vi "Antenna_in.vi"(6 "Store":T1=enum."in_up", 8 "error in (no error)":errorcluster, 10 "Waveform in":waveform(dbl), 11 "RFID system in":refnum<class "RFID system.lvclass">) -> (0 "error out":errorcluster, 2 "Waveform out":waveform(dbl), 3 "RFID system out":refnum<class "RFID system.lvclass">)   [LabVIEW 2019, in "RFID system.lvclass"]
uses:
  RFID system.lvclass
  TypeDef/Store.ctl
  <vilib>/measure/macond.llb/IIR Filter for 1 Chan.vi
  <vilib>/measure/NI_MAPro.lvlib
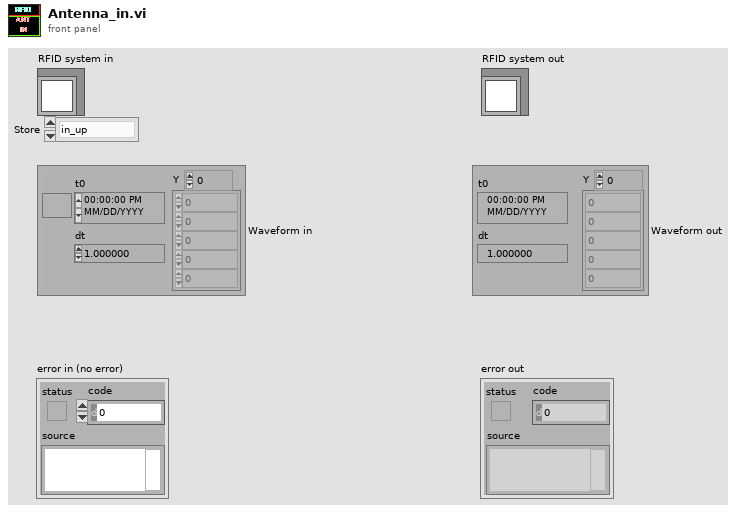
[diagram p1: front panel]
types:
  T1 = typedef "Store.ctl" = enum16{"envelope", "noise", "demSubCar", "CH_frame", "Decode", "demodulate", "in", "out", "sum", "subCarrier", "frame", "command", "encode", "modulate", "encode_UP", "modulate_up", "demod_up", "envelop_up", "sum_up", "out_up", "in_up"}
  T2 = cluster{"Topology":enum16{"Off", "Butterworth", "Chebyshev", "Inverse Chebyshev", "Elliptic", "Bessel"}, "Type":enum16{"Lowpass", "Highpass", "Bandpass", "Bandstop"}, "Order":i32, "Lower Fc":dbl, "Upper Fc":dbl, "PB Ripple":dbl, "SB Attenuation":dbl}
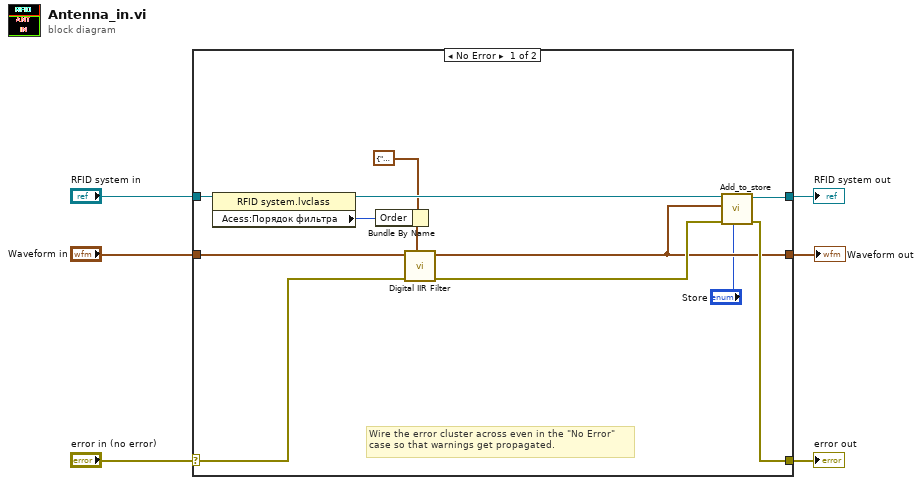
[diagram p0: block diagram]
diagram:
  n1 = case shown="No Error" "error in (no error)" {
    selector: "error in (no error)" -> [w17 w21]
    tunnel: [w13 w21] -> w5
    tunnel: [w15 w20] -> w3
    tunnel: "RFID system in" -> [w16 w20]
    tunnel: "Waveform in" -> [w18 w19]
    tunnel: [w12 w19] -> w1
    frame No Error {
      # "Wire the error cluster across even in the \"No Error\"\ncase so that warnings get propagated."
      n2 = property class="RFID system.lvclass"(reference=w16) -> (reference out=w10:refnum<class "RFID system.lvclass">, "Acess:Порядок фильтра"=w7:i64)  [unwired: 1 in, 1 out]
      n3 = Bundle By Name(cluster=T2 {"Topology"=enum."Butterworth", "Type"=enum."Bandpass", "Order"=3, "Lower Fc"=2000.0, "Upper Fc"=22000.0, "PB Ripple"=1.0, "SB Attenuation"=60.0} ("IIR filter specifications"), "Order"=w7) -> (w8:T2)
      n4 = call-poly <vilib>:"Digital IIR Filter.vi"("IIR filter specifications"=w8, "error in (no error)"=w17, "signal in"=w18) -> ("error out"=w14:errorcluster, "signal out"=w12:waveform(dbl))  [unwired: 6 in, 1 out]
      n5 = call "Add_to_store.vi"("Store"="Store", "error in (no error)"=w14, "Waveform"=w12, "RFID system in"=w10) -> ("error out"=w13:errorcluster, "RFID system out"=w15:refnum<class "RFID system.lvclass">)  [unwired: 6 in]
    }
    frame Error {
    }
  }
  "error out" <- w5
  "RFID system out" <- w3
  "Waveform out" <- w1
